vi "(Incomplete) Gamma Function.vi"   [LabVIEW 2024, in "NI_Gmath.lvlib"]
doc: "<p>Evaluates the gamma function and regularized incomplete gamma function. You must <a href=\"nihelplauncher://docs/csh?context=lvcore_lvhowto_selectingdefaultinstpolyvi\">manually select the polymorphic instance</a> you want to use.</p>"
uses:
  NI_Gmath.lvlib
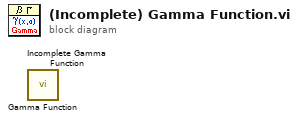
[diagram p0: block diagram]
diagram:
  n1 = call "Gamma Function.vi"() -> ()  [unwired: 11 in, 1 out]
  n2 = call "Incomplete Gamma Function.vi"() -> ()  [unwired: 11 in, 1 out]
